vi "Run RT VI in project.vi"(4 "Run Time":u32, 6 "configuration file path":path, 7 "ip address":string, 8 "error in (no error)":errorcluster, 9 "target alias":string, 10 "vi name":string, 11 "Project Path":path) -> (0 "error out":errorcluster, 1 "invoked VI error out":errorcluster)   [LabVIEW 2014]
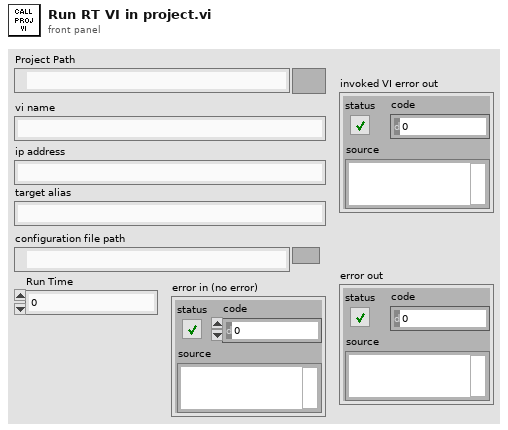
[diagram p1: front panel]
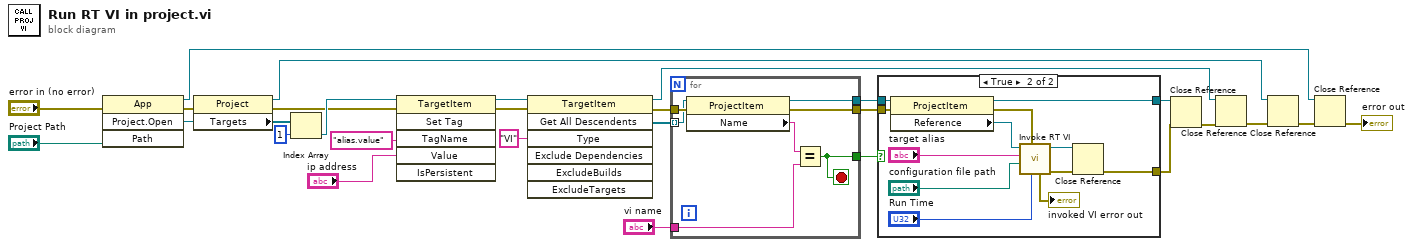
[diagram p0: block diagram]
diagram:
  n1 = invoke class="App" method="Project.Open"(error in="error in (no error)", "Path"="Project Path") -> (reference out=w10:refnum<vi>, error out=w27:errorcluster, "Project:Open"=w28:refnum<vi>)  [unwired: 2 in, 1 out]
  n2 = property class="Project"(reference=w28, error in=w27) -> (reference out=w12:refnum<vi>, error out=w4:errorcluster, "Targets"=w26:refnum<vi>[])
  n3 = Index Array(array=w26, index=1) -> (element=w7:refnum<vi>)
  n4 = invoke class="TargetItem" method="Set Tag"(reference=w7, error in=w4, "TagName"="alias.value" ("Tag Name"), "Value"="ip address") -> (reference out=w2:refnum<vi>, error out=w3:errorcluster)  [unwired: 2 in, 4 out]
  n5 = invoke class="TargetItem" method="Get All Descendents"(reference=w2, error in=w3, "Type"="VI") -> (reference out=w14:refnum<vi>, error out=w23:errorcluster, "All Descendents"=w24:refnum<vi>[])  [unwired: 4 in, 4 out]
  n6 = for {
    tunnel: w24 -> [w29] mode=indexing
    tunnel: w23 -> [w35]
    tunnel: "vi name" -> [w34]
    tunnel: [w33] -> w20
    tunnel: [w32] -> w19
    tunnel: [w31] -> w18
    stop <- w31 stop-if-true
    n7 = property class="ProjectItem"(reference=w29, error in=w35) -> (reference out=w33:refnum<vi>, error out=w32:errorcluster, "Name"=w30:string)
    n8 = Equal?(x=w30, y=w34) -> (x = y?=w31:bool)
  }
  n9 = case shown="True" w18 {
    tunnel: w20 -> [w36 w49]
    tunnel: w19 -> [w37 w48]
    tunnel: [w37 w47] -> w17
    tunnel: [w36 w46] -> w16
    frame False {
    }
    frame True {
      n10 = property class="ProjectItem"(reference=w49, error in=w48) -> (reference out=w46:refnum<vi>, error out=w39:errorcluster, "Reference"=w45:refnum<vi>)
      n11 = call "Invoke RT VI.vi"("Run Time"="Run Time", "error in (no error)"=w39, "configuration file path"="configuration file path", "target alias"="target alias", "reference"=w45) -> ("error out"=w41:errorcluster, "reference out"=w40:refnum<vi>, "invoked VI error out"=→"invoked VI error out":errorcluster)  [unwired: 4 in]
      n12 = Close Reference(reference=w40, error in (no error)=w41) -> (error out=w47:errorcluster)
    }
  }
  n13 = Close Reference(reference=w16, error in (no error)=w17) -> (error out=w15:errorcluster)
  n14 = Close Reference(reference=w14, error in (no error)=w15) -> (error out=w13:errorcluster)
  n15 = Close Reference(reference=w12, error in (no error)=w13) -> (error out=w11:errorcluster)
  n16 = Close Reference(reference=w10, error in (no error)=w11) -> (error out=→"error out":errorcluster)
